vi "network_test.vi"() -> ()   [LabVIEW 2021]
uses:
  FPGA/reciver params.ctl
panel:
  in  "stop":bool
  out "data out":string
  in  "ip_dest":string="10.120.32.48"
  out "*(type *) &x":T1(ring)
  out "p param":T2={"min PW (fft cycels)"=5, "max PW (fft cycels)"=500, "max gap (fft cycels)"=1, "detection bar (liniar amp)"=1000000.0, "peak detect"=FALSE}
  out "u param":cluster{dbl, dbl, dbl, u8}
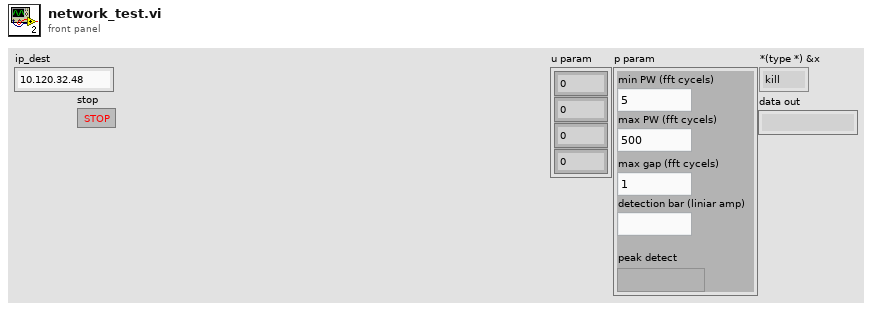
[diagram p1: front panel]
types:
  T1 = enum16{"kill", "turn off", "wait", "run", "turn on"}
  T2 = typedef "reciver params.ctl" = cluster{"min PW (fft cycels)":u16, "max PW (fft cycels)":u16, "max gap (fft cycels)":u8, "detection bar (liniar amp)":fxp<+,64,63>, "peak detect":bool}
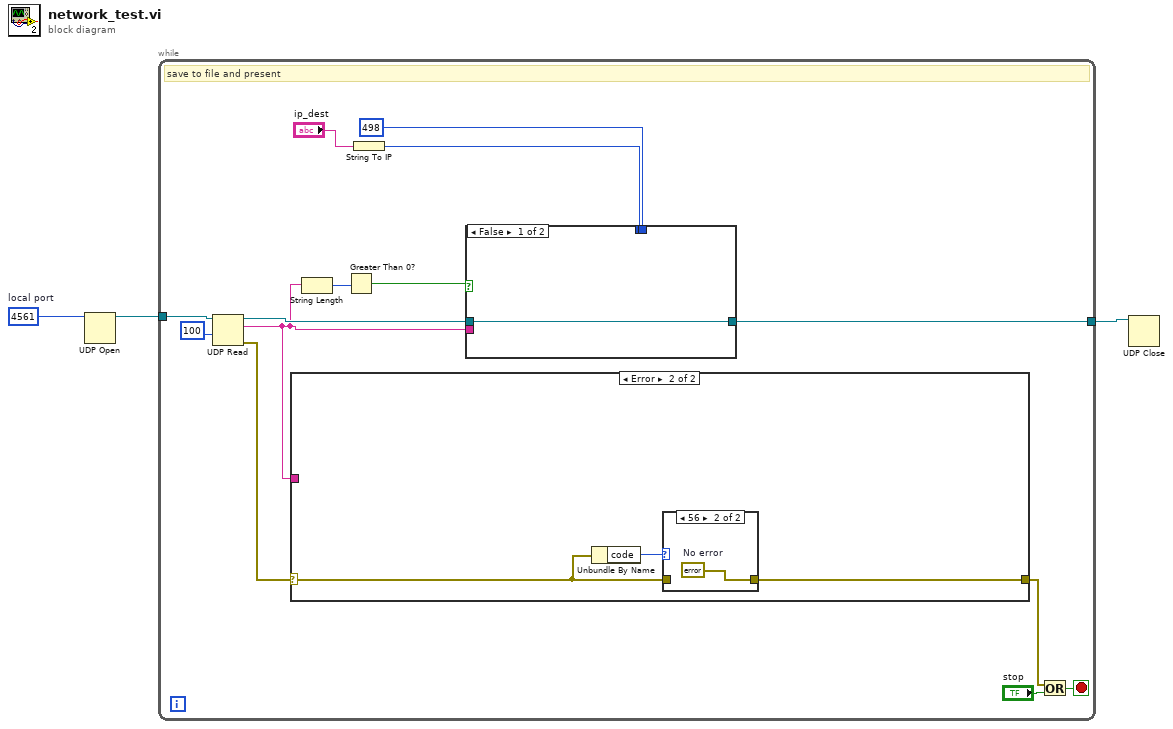
[diagram p0: block diagram]
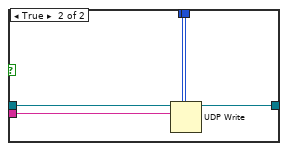
[diagram p2: hidden frame]
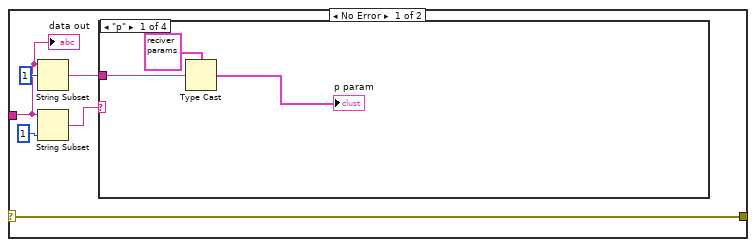
[diagram p3: hidden frame]
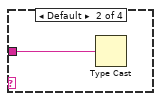
[diagram p4: hidden frame]
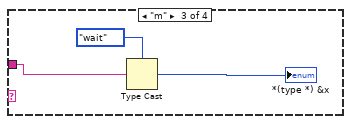
[diagram p5: hidden frame]
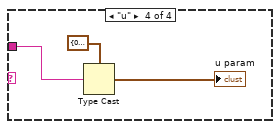
[diagram p6: hidden frame]
diagram:
  w3 = u16 4561  # local port
  n1 = UDP Open(11:w3) -> (port=w2:refnum<k16>)  [unwired: 4 in, 2 out]
  n2 = while {
    tunnel: [w14] -> w1
    tunnel: w2 -> [w13]
    stop <- w4 stop-if-true
    # "save to file and present"
    n3 = UDP Read(connection ID=w13, timeout ms (25000)=100) -> (data out=w8:string, error out=w16:errorcluster, 3:w15:refnum<k16>)  [unwired: 1 in, 3 out]
    n4 = case shown="Error" w16 {
      selector: w16 -> [w29 w41]
      tunnel: [w29 w40] -> w6
      tunnel: w8 -> [w24 _]
      frame No Error {
        # "Sender sent data. Update the chart value."
        n5 = String Subset(string=w24, offset (0)=1) -> (substring=w26:string)  [unwired: 1 in]
        n6 = String Subset(string=w24, length (rest)=1 ("length (rest)")) -> (substring=w25:string)  [unwired: 1 in]
        n7 = case shown="\"p\"" w25 {
          tunnel: w26 -> [w32 w33 w36 w39]
          frame "p" {
            n8 = Type Cast(type=T2 {"min PW (fft cycels)"=5, "max PW (fft cycels)"=500, "max gap (fft cycels)"=1, "detection bar (liniar amp)"=1000000.0, "peak detect"=FALSE} ("reciver_params"), x=w32) -> (*(type *) &x=→"p param":T2)
          }
          frame Default {
            n9 = Type Cast(x=w33) -> ()  [unwired: 1 in, 1 out]
          }
          frame "m" {
            n10 = Type Cast(type=T1."wait", x=w36) -> (*(type *) &x=→"*(type *) &x":T1)
          }
          frame "u" {
            n11 = Type Cast(type=cluster{dbl, dbl, dbl, u8} {0.0, 0.0, 0.0, 0}, x=w39) -> (*(type *) &x=→"u param":cluster{dbl, dbl, dbl, u8})
          }
        }
        "data out" <- w24
      }
      frame Error {
        # "Sender did not send data. Ignore timeout error and keep waiting."
        n12 = Unbundle By Name(w41) -> ("code"=w42:i32)
        n13 = case shown="56" w42 {
          tunnel: w41 -> [w43 _]
          tunnel: [w43 w44] -> w40
          frame Default {
          }
          frame 56 {
            w44 = errorcluster {"status"=FALSE, "code"=0, "source"=""}  # No error
          }
        }
      }
    }
    n14 = String Length(string=w8) -> (length=w9:i32)
    n15 = Greater Than 0?(x=w9) -> (x > 0?=w7:bool)
    n16 = String To IP(1:"ip_dest") -> (0:w11:u32)
    n17 = case shown="False" w7 {
      tunnel: w15 -> [w18 w23]
      tunnel: [w18 w22] -> w14
      tunnel: w11 -> [_ w21]
      tunnel: u16 498 ("port or service name") -> [_ w20]
      tunnel: w8 -> [_ w19]
      frame False {
      }
      frame True {
        n18 = UDP Write(address=w21, port or service name=w20, connection ID=w23, data in=w19) -> (3:w22:refnum<k16>)  [unwired: 2 in, 1 out]
      }
    }
    n19 = Or(x=w6, y="stop") -> (x .or. y?=w4:bool)
  }
  n20 = UDP Close(connection ID=w1) -> ()  [unwired: 1 in, 2 out]
